vi "is a.vi"(8 "error in (no error)":errorcluster, 11 "DAQ  in":refnum<class "DAQ .lvclass">) -> (0 "error out":errorcluster, 2 "is a":string, 3 "DAQ  out":refnum<class "DAQ .lvclass">)   [LabVIEW 2016, in "Hardware.lvlib" / "DAQ .lvclass"]
uses:
  DAQ .lvclass
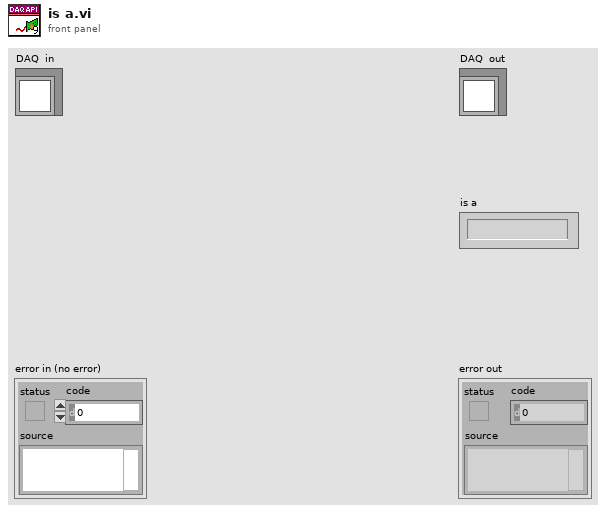
[diagram p1: front panel]
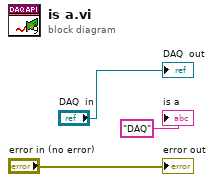
[diagram p0: block diagram]
diagram:
  "error out" <- "error in (no error)"
  "DAQ  out" <- "DAQ  in"
  "is a" <- "DAQ" ("is a")
